vi "AutoRampOnly.vi"() -> ()   [LabVIEW 2012, in "MainProject.lvrbt"]
uses:
  MainProject.lvrbt
  <vilib>/NXT/Hardware/Plugins/Tetrix DC Motor/TetrixDCMotorAddress.ctl
  Drivers/AutoDriverControl.ctl
  FTC 2012 - 2013/Controls/SpeedControl.ctl
  <vilib>/NXT/NXTIO Xnodes/NXTIONodeSubVIs/TETRIX IO Check Battery.vi
  <vilib>/NXT/Dual Mode Library/Waits/Wait_Num(msec).vi
  <vilib>/NXT/NXTIO Xnodes/NXTIONodeSubVIs/TETRIX IO Stop DC Motors.vi
  <vilib>/NXT/Subs/LVHSConnector.ctl
  <vilib>/NXT/NXTIO Xnodes/AddressXNode/NXTIOAddress.xnode
  BlankTemplates/BlankTemplates.lvrbt
  <vilib>/NXT/NXTIO Xnodes/NXTIOXNode/NXTIO.xnode
  <vilib>/NXT/LegoClasses/BrickReference/BrickReference.lvclass
panel:
  out "Enabled":bool
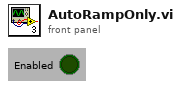
[diagram p1: front panel]
types:
  T1 = typedef "TetrixDCMotorAddress.ctl" = i16
  T2 = typedef "LVHSConnector.ctl" = refnum<class "BrickReference.lvclass">
  T3 = typedef "SpeedControl.ctl" = enum16{"Fast", "Medium", "Slow"}
  T4 = typedef "AutoDriverControl.ctl" = enum16{"Init", "Forward", "Reverse", "Left", "Right", "Brake"}
  T5 = cluster{"TetrixDCMotor":T1, "TetrixDCMotor 2":T1}
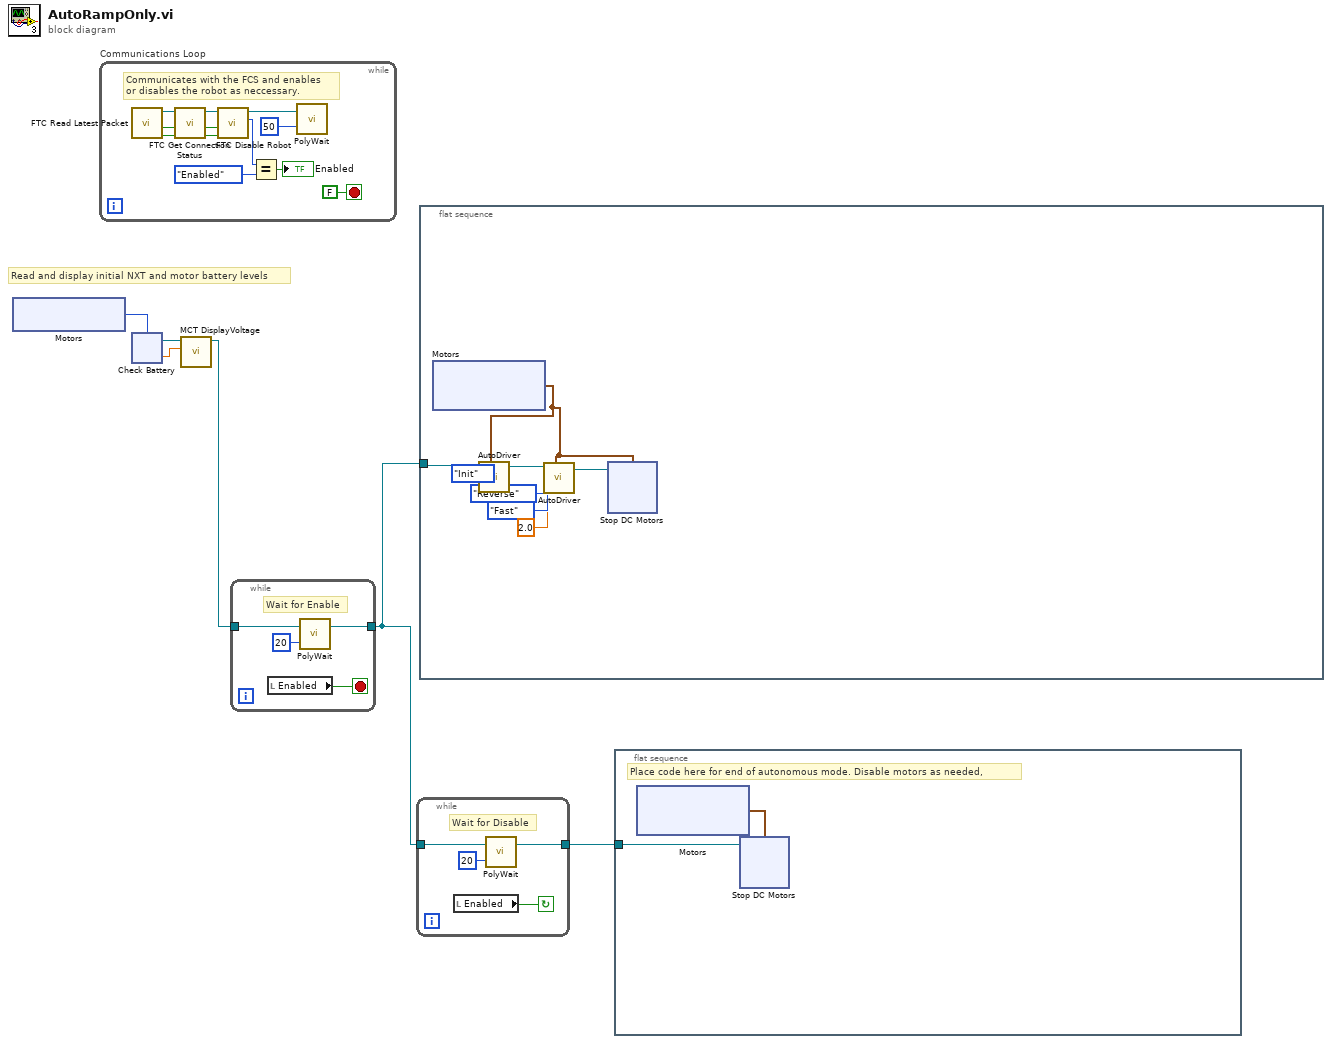
[diagram p0: block diagram]
diagram:
  # "Read and display initial NXT and motor battery levels"
  n1 = xnode "Motors"() -> ("Motor"=w6:T1)
  n2 = while "Communications Loop" {
    stop <- FALSE stop-if-true
    # "Communicates with the FCS and enables \nor disables the robot as neccessary."
    n3 = call <vilib>:"FTC Read Latest Packet.vi"() -> ("Packet Received?"=w16:bool, "Stopped?"=w15:bool, "NXT"=w18:T2)  [unwired: 6 in, 3 out]
    n4 = call <vilib>:"FTC Get Connection Status.vi"("Packet Received?"=w16, "Stopped?"=w15, "NXT"=w18) -> ("Online?"=w7:bool, "Stopped?"=w8:bool, "NXT"=w17:T2)  [unwired: 5 in]
    n5 = call <vilib>:"FTC Disable Robot.vi"("Online?"=w7, "Stopped?"=w8, "NXT"=w17) -> ("Enabled?"=w11:enum16{"Disabled", "Enabled"}, "NXT"=w13:T2)  [unwired: 3 in]
    n6 = Equal?(x=w11, y=enum16{"Disabled", "Enabled"}."Enabled") -> (x = y?=→"Enabled":bool)
    n7 = call-poly <vilib>:"PolyWait.vi"("Time (100 msec)"=u32 50 ("Time (msec)"), "NXT"=w13) -> ()  [unwired: 2 in, 1 out]
  }
  n8 = xnode "Check Battery"("Motors"=w6) -> ("Voltage 1"=w1:sgl, "NXT"=w3:T2)  [unwired: 1 in]
  n9 = call <vilib>:"MCT DisplayVoltage.vi"("Motor Voltage"=w1, "NXT"=w3) -> ("NXT"=w2:T2)  [unwired: 9 in]
  n10 = while {
    tunnel: [w20] -> w5
    tunnel: w2 -> [w19]
    stop <- w21 stop-if-true
    # "Wait for Enable"
    n11 = local read "Enabled"() -> (w21:bool)
    n12 = call-poly <vilib>:"PolyWait.vi"("Time (100 msec)"=u32 20 ("Time (msec)"), "NXT"=w19) -> ("NXT"=w20:T2)  [unwired: 2 in]
  }
  n13 = while {
    tunnel: [w24] -> w4
    tunnel: w5 -> [w23]
    stop <- w25 continue-if-true
    # "Wait for Disable"
    n14 = local read "Enabled"() -> (w25:bool)
    n15 = call-poly <vilib>:"PolyWait.vi"("Time (100 msec)"=u32 20 ("Time (msec)"), "NXT"=w23) -> ("NXT"=w24:T2)  [unwired: 2 in]
  }
  n16 = flat-sequence {
    tunnel: w5 -> [w34]
    frame #0 {
      n17 = xnode "Motors"() -> ("Motor"=w27:cluster{"TetrixDCMotor":T1, "TetrixDCMotor":T1})
      n18 = call "AutoDriver.vi"("NXT In"=w34, "Motors"=w27, "Direction"=AutoDriverControl."Init") -> ("NXT Out"=w32:T2)  [unwired: 5 in]
      n19 = call "AutoDriver.vi"("NXT In"=w32, "Motors"=w27, "Direction"=AutoDriverControl."Reverse", "Speed"=SpeedControl."Fast", "Time (1 sec)"=sgl 2.0) -> ("NXT Out"=w28:T2)  [unwired: 3 in]
      n20 = xnode "Stop DC Motors"("Motors"=w27, "NXT"=w28) -> ()  [unwired: 1 out]
    }
  }
  n21 = flat-sequence {
    tunnel: w4 -> [w44]
    frame #0 {
      # "Place code here for end of autonomous mode. Disable motors as needed,"
      n22 = xnode "Motors"() -> ("Motor"=w43:cluster{"TetrixDCMotor":T1, "TetrixDCMotor":T1})
      n23 = xnode "Stop DC Motors"("Motors"=w43, "NXT"=w44) -> ()  [unwired: 1 out]
    }
  }
